vi "BPM_PROCESSING.vi"(0 "waveform in":waveform(dbl)) -> (1 "output waveform":waveform(dbl), 2 "x*y":dbl)   [LabVIEW 2023]
uses:
  <vilib>/Analysis/3filter.llb/Filter Passband Type.ctl
  <vilib>/Analysis/3filter.llb/Butterworth Filter (DBL).vi
  <vilib>/addons/Time Series Analysis/Series Preprocess.llb/TSA Moving Average (Array).vi
  <vilib>/measure/matone.llb/Extract Single Tone Information 1 Chan.vi
  <vilib>/measure/maresamp.llb/Resample Waveform (single shot).vi
  <vilib>/measure/NI_MAPro.lvlib
  <vilib>/Analysis/NI_AALPro.lvlib
  <vilib>/Analysis/NI_AALBase.lvlib
  <vilib>/addons/_Advanced Signal Processing/NI_AdvSigProcTSA.lvlib
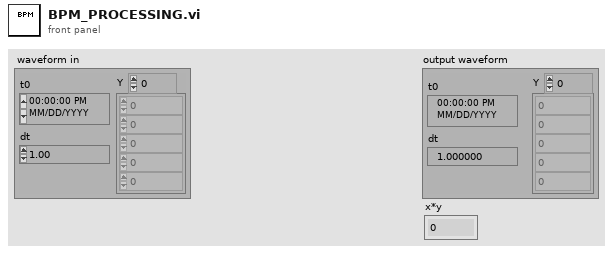
[diagram p1: front panel]
types:
  T1 = typedef "NI_AALBase.lvlib/Filter Passband Type.ctl" = enum32{"Lowpass", "Highpass", "Bandpass", "Bandstop"}
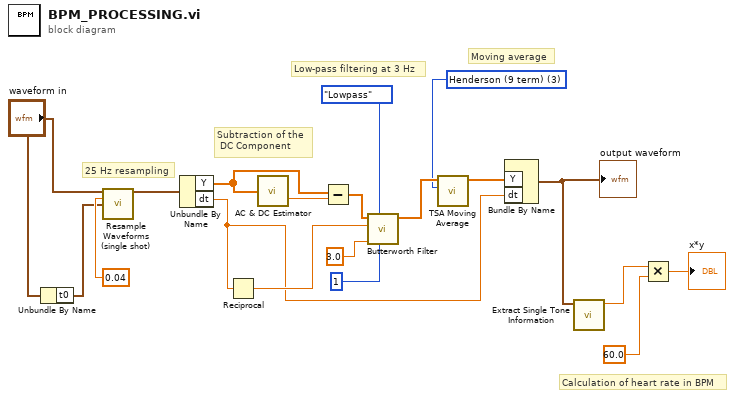
[diagram p0: block diagram]
diagram:
  w10 = 3 items=["Spencer(15 term)"=1, "Henderson (7 term)"=2, "Henderson (9 term)"=3, "Henderson (13 term)"=4, "Henderson (23 term)"=5] ("method")
  # "Calculation of heart rate in BPM"
  # "Moving average"
  # "Low-pass filtering at 3 Hz"
  # "Subtraction of the\n DC Component"
  # "25 Hz resampling"
  n1 = Unbundle By Name("waveform in") -> ("t0"=w18:timestamp)
  n2 = call-poly <vilib>:"Resample Waveforms (single shot).vi"("waveform in"="waveform in", "dt"=0.04, "t0"=w18) -> ("resampled waveform out"=w16:waveform(dbl))  [unwired: 9 in, 3 out]
  n3 = Unbundle By Name(w16) -> ("Y"=w14:dbl[], "dt"=w6:dbl)
  n4 = Reciprocal(x=w6) -> (1/x=w12:dbl)
  n5 = call <vilib>:"AC & DC Estimator.vi"("Signal (V)"=w14) -> ("DC estimate (V)"=w15:dbl)  [unwired: 1 out]
  n6 = Subtract(x=w14, y=w15) -> (x-y=w13:dbl[])
  n7 = call-poly <vilib>:"Butterworth Filter.vi"("order"=1, "filter type"=Filter_Passband_Type."Lowpass", "low cutoff freq: fl"=3.0, "sampling freq: fs"=w12, "X"=w13) -> ("Filtered X"=w11:dbl[])  [unwired: 3 in, 1 out]
  n8 = call-poly <vilib>:"TSA Moving Average.vi"("method"=w10, "Xt"=w11) -> ("Xt out"=w5:dbl[])  [unwired: 8 in, 1 out]
  n9 = Bundle By Name("Y"=w5, "dt"=w6) -> (w4:waveform(dbl))  [unwired: 1 in]
  "output waveform" <- w4
  n10 = call-poly <vilib>:"Extract Single Tone Information.vi"("time signal in"=w4) -> ("detected frequency"=w3:dbl)  [unwired: 5 in, 5 out]
  n11 = Multiply(x=w3, y=60.0) -> (x*y=→"x*y":dbl)
